vi "HeaderBis.vi"(0 "UUTHeader":string, 1 "P/N UUT":string, 2 "Tester HW":string, 3 "DSP SN":string, 4 "Driver S/N":string, 5 "error in":errorcluster, 6 "Product Rev":string, 7 "VR":string, 8 "Approved":string, 10 "POWER SN":string, 11 "Oper.":string, 12 "Revision Param":string, 13 "Tester Software Ver":string) -> (14 "table header":string, 15 "Array":string[][](array[string]), 19 "error out":errorcluster)   [LabVIEW 2017]
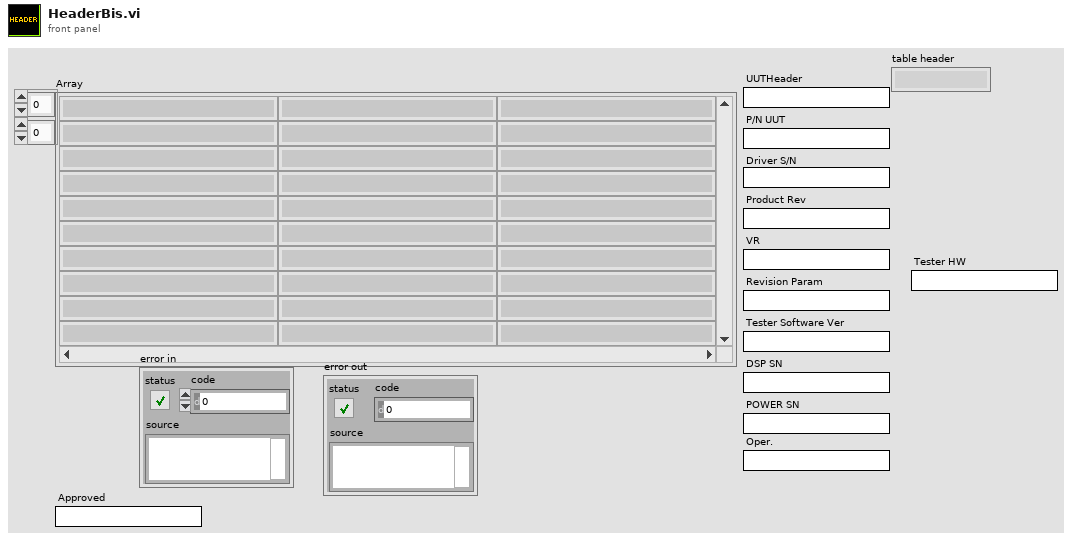
[diagram p1: front panel]
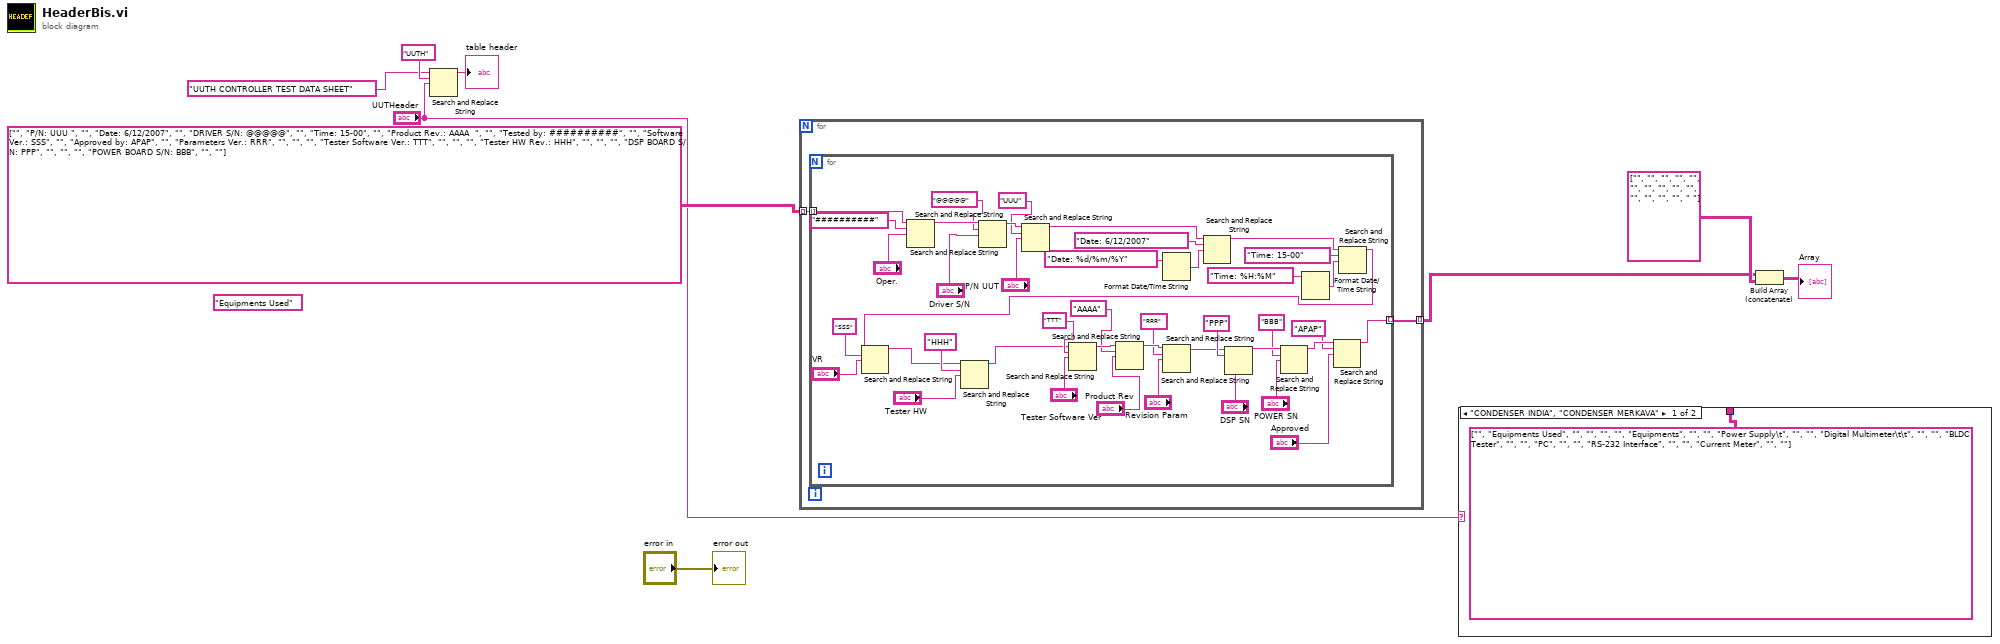
[diagram p0: block diagram]
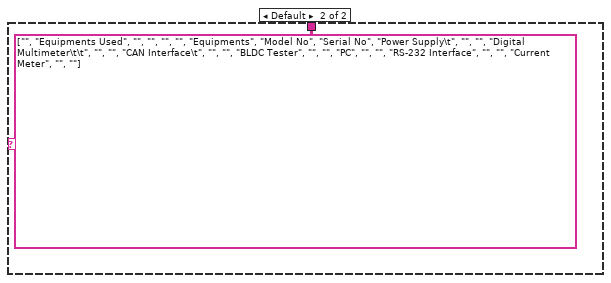
[diagram p2: hidden frame]
diagram:
  (unwired) "Equipments Used"
  n1 = Search and Replace String(input string="UUTH CONTROLLER TEST DATA SHEET", search string="UUTH", replace string="UUTHeader") -> (result string=→"table header":string)  [unwired: 5 in, 3 out]
  n2 = for {
    tunnel: string[][] [["", "P/N: UUU ", "", "Date: 6/12/2007"], ["", "DRIVER S/N: @@@@@", "", "Time: 15-00"], ["", "Product Rev.: AAAA  ", "", "Tested by: ##########"], ["", "Software Ver.: SSS", "", "Approved by: APAP"], ["", "Parameters Ver.: RRR", "", ""], ["", "Tester Software Ver.: TTT", "", ""], ["", "Tester HW Rev.: HHH", "", ""], ["", "DSP BOARD S/N: PPP", "", ""], ["", "POWER BOARD S/N: BBB", "", ""]] -> [w11] mode=indexing
    tunnel: [w10] -> w4 mode=indexing
    n3 = for {
      tunnel: w11 -> [w26] mode=indexing
      tunnel: [w14] -> w10 mode=indexing
      n4 = Search and Replace String(input string=w26, search string="##########" ("source"), replace string="Oper.") -> (result string=w39:string)  [unwired: 5 in, 3 out]
      n5 = Search and Replace String(input string=w39, search string="@@@@@" ("source"), replace string="Driver S/N") -> (result string=w41:string)  [unwired: 5 in, 3 out]
      n6 = Search and Replace String(input string=w41, search string="UUU" ("source"), replace string="P/N UUT") -> (result string=w40:string)  [unwired: 5 in, 3 out]
      n7 = Format Date/Time String(time format string (%c)="Date: %d/%m/%Y") -> (date/time string=w38:string)  [unwired: 2 in]
      n8 = Search and Replace String(input string=w40, search string="Date: 6/12/2007" ("time format string (%c)"), replace string=w38) -> (result string=w49:string)  [unwired: 5 in, 3 out]
      n9 = Format Date/Time String(time format string (%c)="Time: %H:%M") -> (date/time string=w51:string)  [unwired: 2 in]
      n10 = Search and Replace String(input string=w49, search string="Time: 15-00", replace string=w51) -> (result string=w50:string)  [unwired: 5 in, 3 out]
      n11 = Search and Replace String(input string=w50, search string="SSS", replace string="VR") -> (result string=w17:string)  [unwired: 5 in, 3 out]
      n12 = Search and Replace String(input string=w17, search string="HHH", replace string="Tester HW") -> (result string=w16:string)  [unwired: 5 in, 3 out]
      n13 = Search and Replace String(input string=w16, search string="TTT", replace string="Tester Software Ver") -> (result string=w47:string)  [unwired: 5 in, 3 out]
      n14 = Search and Replace String(input string=w47, search string="AAAA", replace string="Product Rev") -> (result string=w53:string)  [unwired: 5 in, 3 out]
      n15 = Search and Replace String(input string=w53, search string="RRR", replace string="Revision Param") -> (result string=w23:string)  [unwired: 5 in, 3 out]
      n16 = Search and Replace String(input string=w23, search string="PPP", replace string="DSP SN") -> (result string=w22:string)  [unwired: 5 in, 3 out]
      n17 = Search and Replace String(input string=w22, search string="BBB", replace string="POWER SN") -> (result string=w15:string)  [unwired: 5 in, 3 out]
      n18 = Search and Replace String(input string=w15, search string="APAP", replace string="Approved") -> (result string=w14:string)  [unwired: 5 in, 3 out]
    }
  }
  n19 = case shown="\"CONDENSER INDIA\", \"CONDENSER MERKAVA\"" "UUTHeader" {
    tunnel: [string[][] [["", "Equipments Used", ""], ["", "", ""], ["Equipments", "", ""], ["Power Supply\t", "", ""], ["Digital Multimeter\t\t", "", ""], ["BLDC Tester", "", ""], ["PC", "", ""], ["RS-232 Interface", "", ""], ["Current Meter", "", ""]] string[][] [["", "Equipments Used", ""], ["", "", ""], ["Equipments", "Model No", "Serial No"], ["Power Supply\t", "", ""], ["Digital Multimeter\t\t", "", ""], ["CAN Interface\t", "", ""], ["BLDC Tester", "", ""], ["PC", "", ""], ["RS-232 Interface", "", ""], ["Current Meter", "", ""]]] -> _
    frame "CONDENSER INDIA", "CONDENSER MERKAVA" {
    }
    frame Default {
    }
  }
  n20 = Build Array (concatenate)(w4, string[][] [["", "", ""], ["", "", ""], ["", "", ""], ["", "", ""], ["", "", " "]]) -> (→"Array":string[][])
  "error out" <- "error in"
